vi "roboRIO v1.0 Get Scaling Constants AI.vi"(8 "error in (no error)":errorcluster, 10 "Channel List":T3) -> (0 "error out":errorcluster, 2 "Scale Constants Array":T1)   [LabVIEW 2021]
uses:
  <vilib>/myRIO/Common/Instrument Driver Framework/myRIO v1.0/AI/typedefs/AI Channels List.ctl
  <vilib>/myRIO/Common/Instrument Driver Framework/myRIO v1.0/AI/typedefs/AI Channels Enum.ctl
  <vilib>/myRIO/Common/Instrument Driver Framework/Utilities/typedefs/Analog Scaling Constants List.ctl
  <vilib>/myRIO/Common/Instrument Driver Framework/Utilities/typedefs/Analog Scaling Constants.ctl
  <vilib>/myRIO/Common/Instrument Driver Framework/roboRIO v1.0/Resource Manager/vis/roboRIO v1.0 Get Scaling Constants.vi
  <vilib>/myRIO/Common/Instrument Driver Framework/Utilities/vis/Parse Scaling Constant Table.vi
  <vilib>/myRIO/Common/Instrument Driver Framework/roboRIO v1.0/Resource Manager/vis/roboRIO v1.0 Scaling Constants Table.vi
  <vilib>/Utility/error.llb/Trim Whitespace.vi
  <vilib>/Utility/error.llb/Error Cluster From Error Code.vi
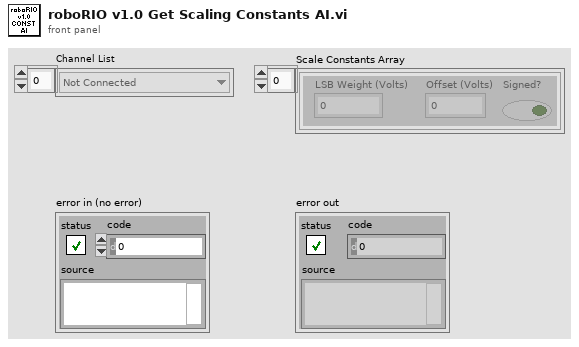
[diagram p1: front panel]
types:
  T1 = typedef "Analog Scaling Constants List.ctl" = T2[]
  T2 = typedef "Analog Scaling Constants.ctl" = cluster{"LSB Weight (Volts)":dbl, "Offset (Volts)":dbl, "Signed?":bool}
  T3 = typedef "AI Channels List.ctl" = T4[]
  T4 = typedef "AI Channels Enum.ctl" = enum16{"Not Connected", "AudioIn/Left", "AudioIn/Right", "C/AI0", "C/AI1", "A/AI0", "A/AI1", "A/AI2", "A/AI3", "A/AI4", "A/AI5", "A/AI6", "A/AI7", "B/AI0", "B/AI1", "B/AI2", "B/AI3", "B/AI4", "B/AI5", "B/AI6", "B/AI7", "AI/AI0", "AI/AI1", "AI/AI2", "AI/AI3", "A/AI0 (DIFF)", "A/AI1 (DIFF)", "A/AI2 (DIFF)", "A/AI3 (DIFF)", "B/AI0 (DIFF)", "B/AI1 (DIFF)", "B/AI2 (DIFF)", "B/AI3 (DIFF)"}
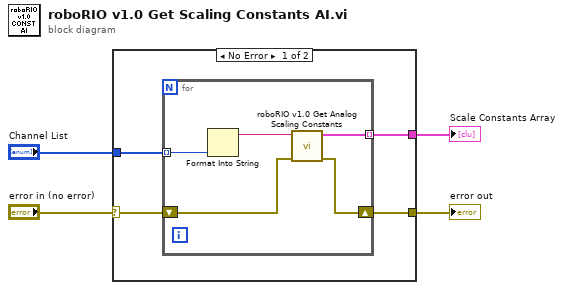
[diagram p0: block diagram]
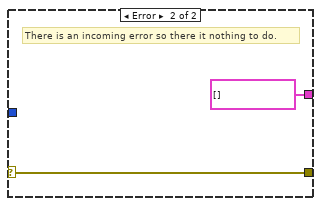
[diagram p2: hidden frame]
diagram:
  n1 = case shown="No Error" "error in (no error)" {
    selector: "error in (no error)" -> [w6 w15]
    tunnel: [w8 w15] -> w4
    tunnel: "Channel List" -> [w7 _]
    tunnel: [w5 T2[] []] -> w1
    frame No Error {
      n2 = for {
        shift-right: [w11] -> w8
        shift-left: w6 -> [w13]
        tunnel: w7 -> [w10] mode=indexing
        tunnel: [w12] -> w5 mode=indexing
        n3 = Format Into String(w10) -> (resulting string=w9:string)  [unwired: 3 in, 1 out]
        n4 = call <vilib>:"roboRIO v1.0 Get Analog Scaling Constants.vi"("error in (no error)"=w13, "Analog Channel Name"=w9) -> ("error out"=w11:errorcluster, "Analog Scaling Constants"=w12:T2)  [unwired: 8 in]
      }
    }
    frame Error {
      # "There is an incoming error so there it nothing to do."
    }
  }
  "error out" <- w4
  "Scale Constants Array" <- w1
